vi "总氮测量数据储存.vi"   [LabVIEW 2016, in "斯坦道总氮.lvlib"]
types:
  T1 = cluster{"时间标识":timestamp, "监测值":sgl, "单位":u16, "数据标识":string, "因子编码":u32, "标样参考值":sgl, "F0":sgl, "F1":sgl, "F2":sgl, "F3":sgl, "F4":sgl, "F5":sgl, "F6":sgl, "F7":sgl, "X":sgl, "温度":sgl, "湿度":sgl, "量程标识":string}
  T2 = enum16{"维护数据", "水样测试", "标样核查", "零点核查", "跨度核查", "空白测试", "平行样测试", "加标回收", "空白校准", "标样校准", "初始化（清洗）"}
  T3 = cluster{"运行模式":enum16{"维护模式", "常规模式", "应急模式", "质控模式"}, "质控频次":enum16{"关闭", "每天", "星期一", "星期二", "星期三", "星期四", "星期五", "星期六", "星期日"}, "空白核查时间":u16, "跨度核查时间":u16, "24H周期设置":bool[]}
  T4 = cluster{"系统时间":timestamp, "工作状态":enum16{"空闲", "水样测试", "标样核查", "零点核查", "跨度核查", "空白测试", "平行样测试", "加标回收", "空白校准", "标样校准", "初始化（清洗）"}, "测量模式":enum16{"待机", "连续模式", "周期模式", "定点模式", "受控模式", "手动模式"}, "告警代码":enum16{"无告警", "缺试剂告警", "缺水样告警", "缺蒸馏水告警", "缺标液告警", "仪表漏液告警", "标定异常告警", "超量程告警", "加热异常", "低试剂预警", "超上限告警", "超下限告警", "仪表内部其他异常", "滴定异常告警", "电极异常告警", "量程切换告警", "参数设置告警", "PH电极电位异常", "电导率电极异常", "浊度光度异常", "溶解氧电极异常", "溶解氧光强异常", "温度异常告警", "PH异常告警", "溶解氧异常告警", "电导率异常告警", "浊度异常告警", "叶绿素异常告警", "藻密度异常告警", "蓝绿藻异常告警", "ORP异常告警", "氨氮异常告警", "清洁刷异常告警", "SD卡异常告警", "蓝牙异常告警", "Wifi异常告警", "流程异常告警"}, "故障代码":enum16{"无故障", "电机故障", "温度故障", "通讯故障", "滴定故障"}, "日志代码":u16, "软件版本":u16, "F0":sgl, "F1":sgl, "F2":sgl, "F3":sgl, "T":sgl, "H":sgl, "id":u16, "flowid":u16, "量程":u16, "总磷控温温度1":sgl, "营养盐控温温度2":sgl, "ADC":sgl}
  T5 = enum16{"空闲", "水样测试", "标样核查", "零点核查", "跨度核查", "空白测试", "平行样测试", "加标回收", "空白校准", "标样校准", "初始化（清洗）"}
  T6 = cluster{"因子编码":u32, "单位":u16, "标样参考值":sgl, "水样数据时间":timestamp, "水样实测值":sgl, "水样数据标识":string, "标样数据时间":timestamp, "标样实测值":sgl, "标样数据标识":string, "空白数据时间":timestamp, "空白实测值":sgl, "空白数据标识":string, "零点核查数据时间":timestamp, "零点核查实测值":sgl, "零点核查数据标识":string, "跨度核查数据时间":timestamp, "跨度核查实测值":sgl, "跨度核查数据标识":string, "加标回收数据时间":timestamp, "加标回收实测值":sgl, "加标回收数据标识":string, "平行样数据时间":timestamp, "平行样实测值":sgl, "平行样数据标识":string, "F0":sgl, "F1":sgl, "F2":sgl, "F3":sgl, "F4":sgl, "F5":sgl, "F6":sgl, "F7":sgl, "温度":sgl, "湿度":sgl, "X值":sgl}
  T7 = cluster{"跨度值":dbl, "零点标准液浓度":dbl, "跨度标准液浓度":dbl, "标准液标准浓度":dbl}
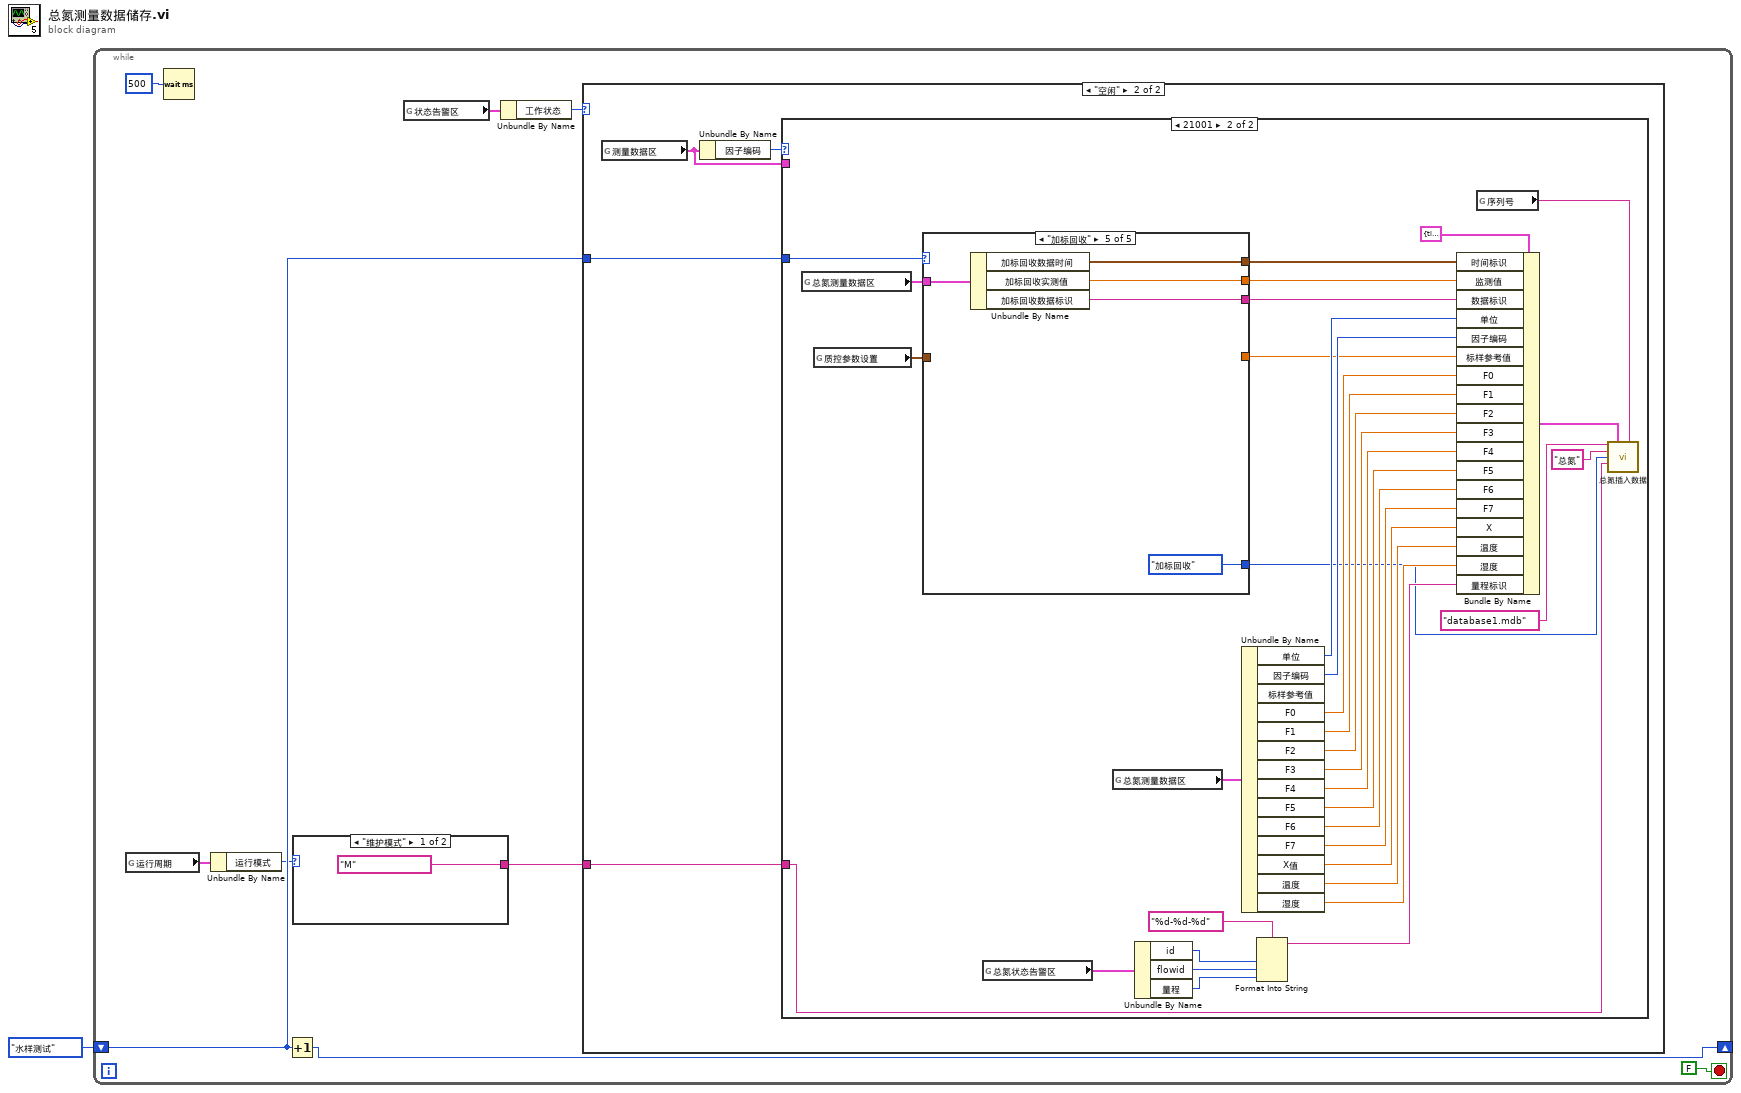
[diagram p0: block diagram]
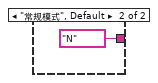
[diagram p2: hidden frame]
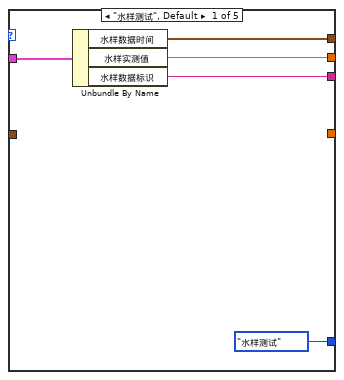
[diagram p5: hidden frame]
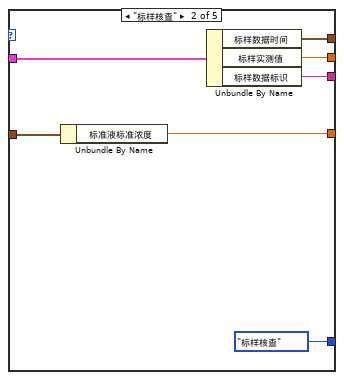
[diagram p6: hidden frame]
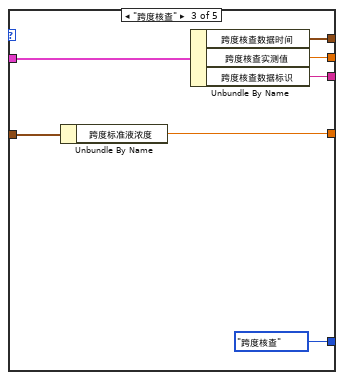
[diagram p7: hidden frame]
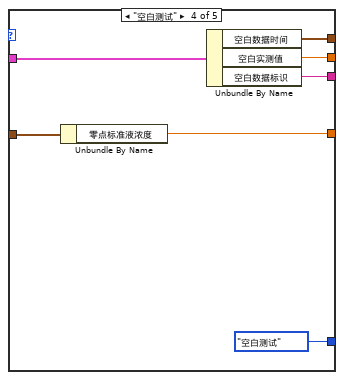
[diagram p8: hidden frame]
diagram:
  n1 = while {
    shift-right: [w6] -> _
    shift-left: enum16{"水样测试", "标样核查", "跨度核查", "空白测试", "加标回收"}."水样测试" ("测量模式") -> [w5]
    stop <- FALSE stop-if-true
    n2 = global read "总氮断电保存全局变量.vi" "运行周期"() -> (w3:T3)
    n3 = Wait (ms)(milliseconds to wait=u32 500 ("等待时间（毫秒）")) -> ()  [unwired: 1 out]
    n4 = Unbundle By Name(w3) -> ("运行模式"=w2:enum16{"维护模式", "常规模式", "应急模式", "质控模式"})
    n5 = Increment(x=w5) -> (x+1=w6:enum16{"水样测试", "标样核查", "跨度核查", "空白测试", "加标回收"})
    n6 = case shown="\"维护模式\"" w2 {
      tunnel: ["M" ("数据标记表") "N" ("数据标记表")] -> w7
      frame "维护模式" {
      }
      frame "常规模式", Default {
      }
    }
    n7 = global read "VAR总氮全局变量.vi" "状态告警区"() -> (w4:T4)
    n8 = Unbundle By Name(w4) -> ("工作状态"=w8:T5)
    n9 = case shown="\"空闲\"" w8 {
      tunnel: w7 -> [_ w14]
      tunnel: w5 -> [_ w13]
      frame Default {
      }
      frame "空闲" {
        n10 = global read "VAR总氮全局变量.vi" "测量数据区"() -> (w16:T6)
        n11 = Unbundle By Name(w16) -> ("因子编码"=w15:u32)
        n12 = case shown="21001" w15 {
          tunnel: w16 -> [_ _]
          tunnel: w14 -> [_ w21]
          tunnel: w13 -> [_ w20]
          frame Default {
          }
          frame 21001 {
            n13 = global read "VAR总氮全局变量.vi" "总氮测量数据区"() -> (w49:T6)
            n14 = global read "总氮断电保存全局变量.vi" "质控参数设置"() -> (w18:T7)
            n15 = case shown="\"加标回收\"" w20 {
              tunnel: w49 -> [w55 w62 w69 w76 w81]
              tunnel: [w54 w61 w68 w75 w80] -> w25
              tunnel: [w53 w60 w67 w74 w79] -> w26
              tunnel: [w52 w59 w66 w73 w78] -> w27
              tunnel: [T2."水样测试" ("测量模式") T2."标样核查" ("测量模式") T2."跨度核查" ("测量模式") T2."空白测试" ("测量模式") T2."加标回收" ("测量模式")] -> w24
              tunnel: w18 -> [_ w57 w64 w71 _]
              tunnel: [_ w56 w63 w70 _] -> w17
              frame "水样测试", Default {
                n16 = Unbundle By Name(w55) -> ("水样数据时间"=w54:timestamp, "水样实测值"=w53:sgl, "水样数据标识"=w52:string)
              }
              frame "标样核查" {
                n17 = Unbundle By Name(w57) -> ("标准液标准浓度"=w56:dbl)
                n18 = Unbundle By Name(w62) -> ("标样数据时间"=w61:timestamp, "标样实测值"=w60:sgl, "标样数据标识"=w59:string)
              }
              frame "跨度核查" {
                n19 = Unbundle By Name(w64) -> ("跨度标准液浓度"=w63:dbl)
                n20 = Unbundle By Name(w69) -> ("跨度核查数据时间"=w68:timestamp, "跨度核查实测值"=w67:sgl, "跨度核查数据标识"=w66:string)
              }
              frame "空白测试" {
                n21 = Unbundle By Name(w71) -> ("零点标准液浓度"=w70:dbl)
                n22 = Unbundle By Name(w76) -> ("空白数据时间"=w75:timestamp, "空白实测值"=w74:sgl, "空白数据标识"=w73:string)
              }
              frame "加标回收" {
                n23 = Unbundle By Name(w81) -> ("加标回收数据时间"=w80:timestamp, "加标回收实测值"=w79:sgl, "加标回收数据标识"=w78:string)
              }
            }
            n24 = global read "VAR总氮全局变量.vi" "总氮状态告警区"() -> (w19:T4)
            n25 = global read "VAR总氮全局变量.vi" "总氮测量数据区"() -> (w32:T6)
            n26 = Unbundle By Name(w19) -> ("id"=w50:u16, "flowid"=w34:u16, "量程"=w33:u16)
            n27 = Unbundle By Name(w32) -> ("单位"=w48:u16, "因子编码"=w47:u32, "F0"=w46:sgl, "F1"=w45:sgl, "F2"=w44:sgl, "F3"=w43:sgl, "F4"=w42:sgl, "F5"=w41:sgl, "F6"=w40:sgl, "F7"=w39:sgl, "X值"=w38:sgl, "温度"=w37:sgl, "湿度"=w36:sgl)  [unwired: 1 out]
            n28 = Format Into String(format string="%d-%d-%d" ("格式字符串"), w50, w34, w33) -> (resulting string=w35:string)  [unwired: 2 in, 1 out]
            n29 = Bundle By Name(cluster=T1 {"时间标识"=timestamp(0 s since 1904-01-01), "监测值"=0.0, "单位"=0, "数据标识"="", "因子编码"=0, "标样参考值"=0.0, "F0"=0.0, "F1"=0.0, "F2"=0.0, "F3"=0.0, "F4"=0.0, "F5"=0.0, "F6"=0.0, "F7"=0.0, "X"=0.0, "温度"=0.0, "湿度"=0.0, "量程标识"=""} ("data"), "时间标识"=w25, "监测值"=w26, "数据标识"=w27, "单位"=w48, "因子编码"=w47, "标样参考值"=w17, "F0"=w46, "F1"=w45, "F2"=w44, "F3"=w43, "F4"=w42, "F5"=w41, "F6"=w40, "F7"=w39, "X"=w38, "温度"=w37, "湿度"=w36, "量程标识"=w35) -> (w29:T1)
            n30 = global read "VAR总氮全局变量.vi" "序列号"() -> (w28:string)
            n31 = call "总氮插入数据.vi"("database"="database1.mdb", "data"=w29, "SN"=w28, "table"="总氮", "测量模式"=w24, "数据标记表"=w21) -> ()  [unwired: 9 in, 1 out]
          }
        }
      }
    }
  }
